vi "Test Copy.vi"(8 "error in (no error)":errorcluster, 11 "Test Case In":refnum<class "01_Image.lvclass">) -> (0 "error out":errorcluster, 3 "Test Case Out":refnum<class "01_Image.lvclass">)   [LabVIEW 2020, in "test.lvlib" / "01_Image.lvclass"]
uses:
  01_Image.lvclass
  C:/Program Files (x86)/National Instruments/LabVIEW 2026/vi.lib/Astemes/LUnit/Test Case.lvclass
  common/Image Size (Integer).ctl
  image/ARGB Colour.ctl
  <vilib>/Astemes/LUnit/Test Case.lvclass/Test Case.ctl
  b8792e11-8542-432e-a0d5-9a7d61cf02c7.vi
  image/New Image (ARGB Preallocated).vi
  image/New Image (Greyscale Preallocated).vi
  image/Copy Image (Greyscale).vi
  4993e8ee-a06a-463a-9684-69129f64d5ce.vi
  image/Copy Image (ARGB).vi
  b39dd01c-c990-4813-b992-e0f28e57d61a.vi
  image/Copy Image (ARGB with Greyscale Mask).vi
  547d0f42-e6d8-4a09-97b6-da1091ed9acb.vi
  image/Copy Image (Greyscale with Mask).vi
  ad9f36d4-cc3b-401b-ad87-e6b842f4a90a.vi
  image/Copy Image (ARGB with ARGB Mask).vi
  53ef6583-9edd-4501-a958-4adbe55cf346.vi
  image/New Image (ARGB Preallocated).vi/3321fa97-f432-4e1e-8db9-a0df79aed21b.vi
  image/ARGB Colour to U32 Pixel Value.vi
  image/New Image (Greyscale Preallocated).vi/6598b9e0-8a08-46f5-91fd-ca1b87217137.vi
  image/Copy Image (Greyscale).vi/c92252ab-1097-45af-a449-7a3c8cf05290.vi
  <vilib>/Astemes/LUnit/Core/LUnit Test Case/Private/Append Pass Result.vi
  <vilib>/Astemes/LUnit/Core/LUnit Test Case/Private/Append Fail Result.vi
  4993e8ee-a06a-463a-9684-69129f64d5ce.vi/9c5d11cd-9439-4240-a1ee-d9baace9c924.vi
  image/Copy Image (ARGB).vi/d58821cd-5760-454c-8714-6bb79b1811ae.vi
  b39dd01c-c990-4813-b992-e0f28e57d61a.vi/9c5d11cd-9439-4240-a1ee-d9baace9c924.vi
  image/Copy Image (ARGB with Greyscale Mask).vi/327a14ae-2acc-4952-87c0-fab6c3cd3da3.vi
  547d0f42-e6d8-4a09-97b6-da1091ed9acb.vi/9c5d11cd-9439-4240-a1ee-d9baace9c924.vi
  image/Copy Image (Greyscale with Mask).vi/1519c485-f8d8-4564-b4f6-4c035770646f.vi
  ad9f36d4-cc3b-401b-ad87-e6b842f4a90a.vi/9c5d11cd-9439-4240-a1ee-d9baace9c924.vi
  image/Copy Image (ARGB with ARGB Mask).vi/3b1fb24f-4521-4d3d-a8b9-ed3d08148c99.vi
  53ef6583-9edd-4501-a958-4adbe55cf346.vi/9c5d11cd-9439-4240-a1ee-d9baace9c924.vi
  <vilib>/Astemes/LUnit/Core/LUnit Test Case/Private/Run In UI.vi
  <vilib>/Utility/error.llb/Clear Errors.vi
  <vilib>/Utility/error.llb/Error Cluster From Error Code.vi
  image/image.lvlib
  common/common.lvlib
  <vilib>/Astemes/LUnit/Test Case.lvclass
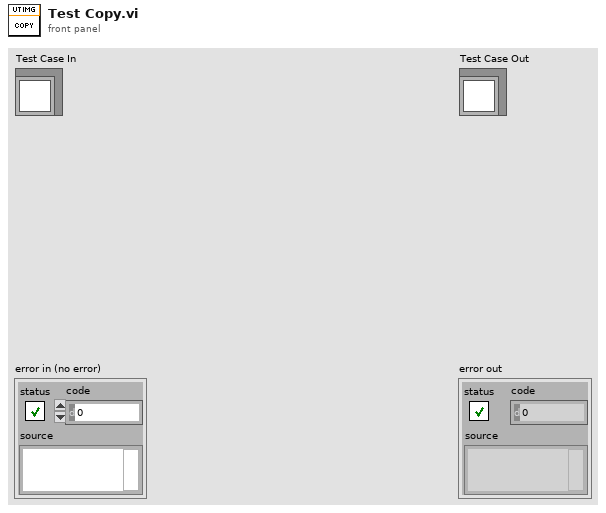
[diagram p1: front panel]
types:
  T1 = typedef "image.lvlib/ARGB Colour.ctl" = cluster{"Alpha":u8, "RGB":u32}
  T2 = typedef "common.lvlib/Image Size (Integer).ctl" = cluster{"Width":u16, "Height":u16}
  T3 = enum16{"ARGB", "Greyscale", "ARGB with Greyscale Mask", "ARGB with ARGB Mask", "Greyscale with Mask"}
  T4 = typedef "image.lvlib/ARGB Image.ctl" = refnum<data-value>
  T5 = typedef "image.lvlib/Greyscale Image.ctl" = refnum<data-value>
  T6 = enum16{"ARGB", "Greyscale", "ARGB with Greyscale Mask", "ARGB with ARGB Mask", "Greyscale with Mask"}[]
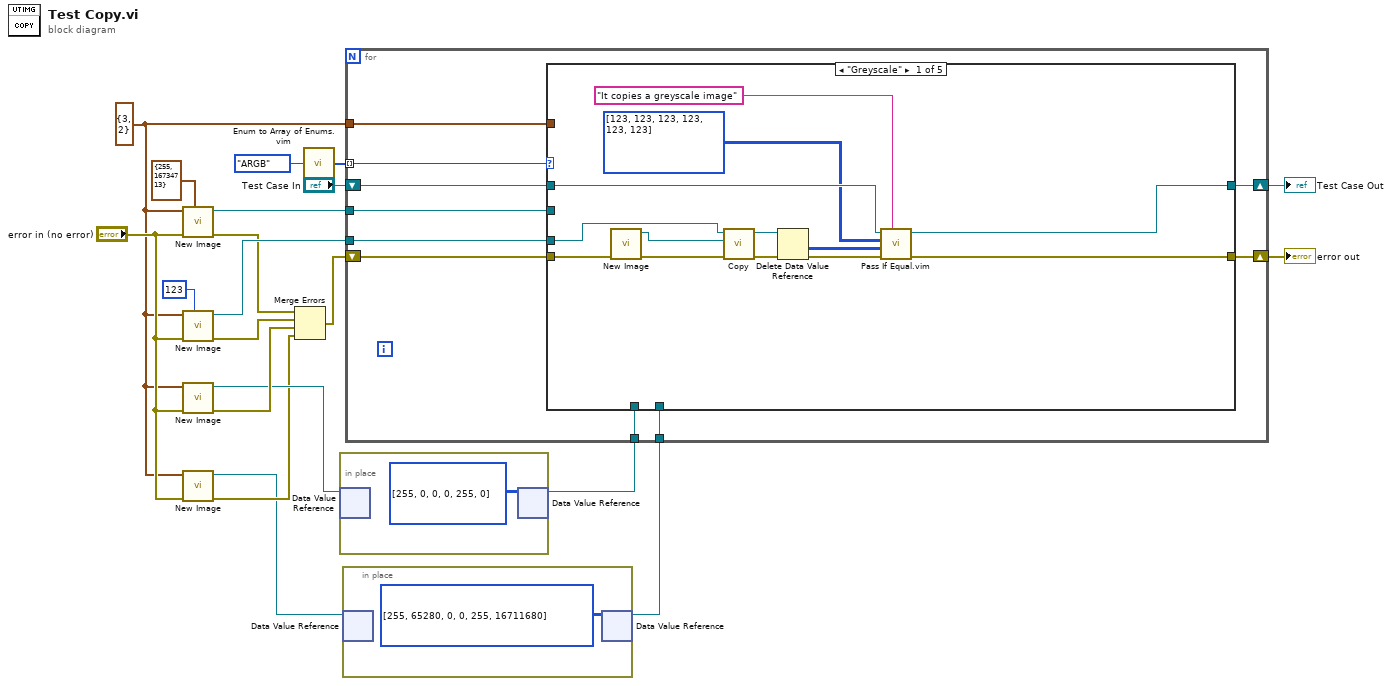
[diagram p0: block diagram]
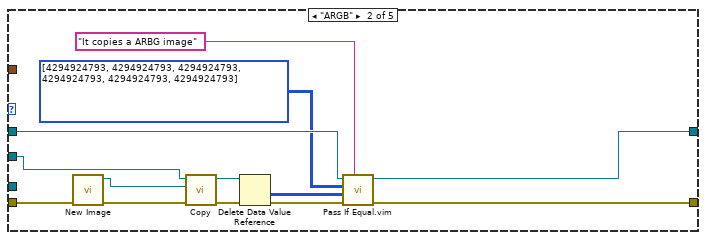
[diagram p2: hidden frame]
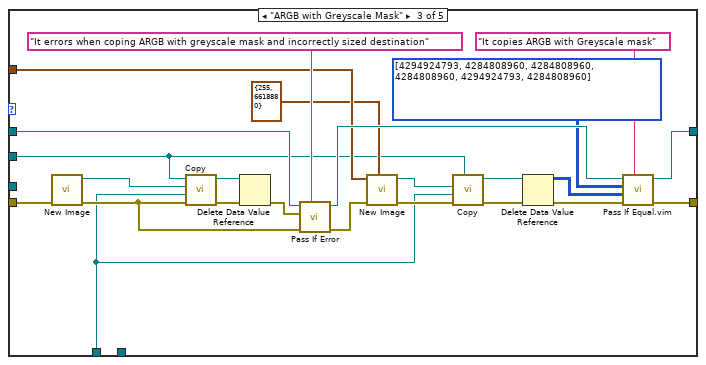
[diagram p3: hidden frame]
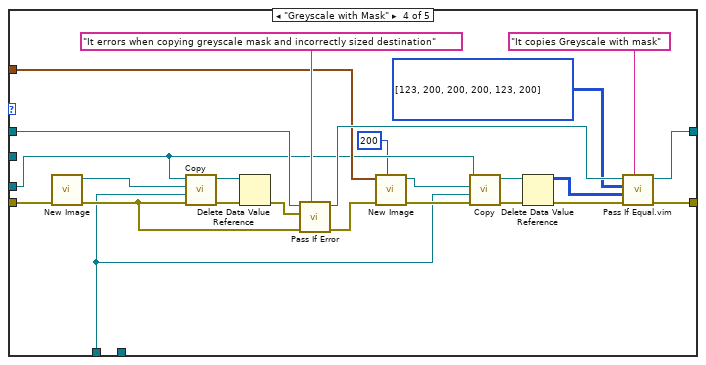
[diagram p4: hidden frame]
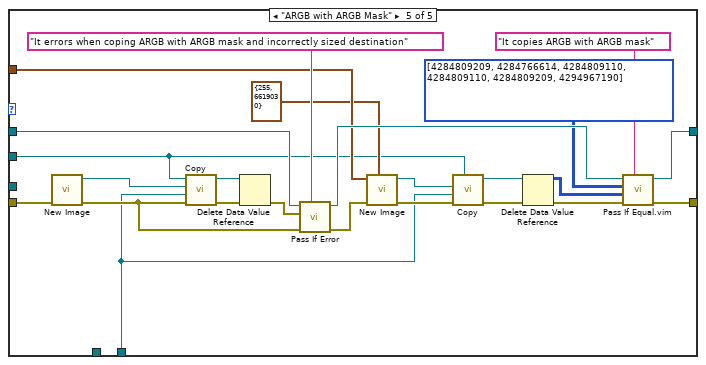
[diagram p5: hidden frame]
diagram:
  w4 = T2 {"Width"=3, "Height"=2} ("Preallocated Image Size (Default: 0,0)")
  n1 = call-poly "New Image.vi"("Colour (Default: Black)"=T1 {"Alpha"=255, "RGB"=16734713}, "error in (no error)"="error in (no error)", "Preallocated Image Size (Default: 0,0)"=w4) -> ("error out"=w13:errorcluster, "ARGB Image"=w14:T4)  [unwired: 7 in]
  n2 = call-poly "New Image.vi"("Value (Default: 0)"=u8 123, "error in (no error)"="error in (no error)", "Preallocated Image Size (Default 0,0)"=w4) -> ("error out"=w12:errorcluster, "Greyscale Image"=w15:T5)  [unwired: 7 in]
  n3 = call-poly "New Image.vi"("error in (no error)"="error in (no error)", "Preallocated Image Size (Default 0,0)"=w4) -> ("error out"=w8:errorcluster, "Greyscale Image"=w7:T5)  [unwired: 8 in]
  n4 = call-poly "New Image.vi"("error in (no error)"="error in (no error)", "Preallocated Image Size (Default: 0,0)"=w4) -> ("error out"=w3:errorcluster, "ARGB Image"=w2:T4)  [unwired: 8 in]
  n5 = Merge Errors(w13, w12, w8, w3) -> (w11:errorcluster)
  n6 = call "Enum to Array of Enums.vim"("enum"=T3."ARGB") -> ("array of enums"=w16:T6)
  n7 = in-place {
    n8 = in-place-dvr #1(w7) -> ()  [unwired: 2 out]
    n9 = in-place-dvr #1(u8[][] [[255, 0, 0], [0, 255, 0]] ("data value")) -> (w6:T5)  [unwired: 1 out]
  }
  n10 = in-place {
    n11 = in-place-dvr #2(w2) -> ()  [unwired: 2 out]
    n12 = in-place-dvr #2(u32[][] [[255, 65280, 0], [0, 255, 16711680]] ("data value")) -> (w1:T4)  [unwired: 1 out]
  }
  n13 = for {
    shift-right: [w31] -> w19
    shift-left: "Test Case In" -> [w32]
    shift-right: [w29] -> w18
    shift-left: w11 -> [w30]
    tunnel: w16 -> [w28] mode=indexing
    tunnel: w15 -> [w27]
    tunnel: w14 -> [w26]
    tunnel: w6 -> [w25]
    tunnel: w4 -> [w24]
    tunnel: w1 -> [w23]
    n14 = case shown="\"Greyscale\"" w28 {
      tunnel: w32 -> [w45 w58 w74 w98 w122]
      tunnel: [w44 w57 w82 w106 w130] -> w31
      tunnel: w30 -> [w40 w54 w79 w103 w127]
      tunnel: [w43 w56 w81 w105 w129] -> w29
      tunnel: w27 -> [w42 _ _ w84 _]
      tunnel: w26 -> [_ w47 w63 _ w112]
      tunnel: w25 -> [_ _ w64 w89 _]
      tunnel: w24 -> [_ _ w66 w90 w114]
      tunnel: w23 -> [_ _ _ _ w109]
      frame "Greyscale" {
        n15 = call-poly "New Image.vi"("error in (no error)"=w40) -> ("error out"=w39:errorcluster, "Greyscale Image"=w38:T5)  [unwired: 9 in]
        n16 = call-poly "Copy.vi"("error in (no error)"=w39, "Greyscale Image Destination in"=w38, "Greyscale Image Source in"=w42) -> ("error out"=w41:errorcluster, "Greyscale Image Destination"=w36:T5)  [unwired: 7 in]
        n17 = Delete Data Value Reference(data value reference=w36, error in=w41) -> (data value=w35:u8[][], error out=w37:errorcluster)
        n18 = call "Pass If Equal.vim"("Description"="It copies a greyscale image", "error in (no error)"=w37, "Actual"=w35, "Expected"=u8[][] [[123, 123, 123], [123, 123, 123]] ("data value"), "LUnit Test Case In"=w45) -> ("error out"=w43:errorcluster, "LUnit Test Case Out"=w44:refnum<class "01_Image.lvclass">)  [unwired: 5 in]
      }
      frame "ARGB" {
        n19 = call-poly "New Image.vi"("error in (no error)"=w54) -> ("error out"=w53:errorcluster, "ARGB Image"=w52:T4)  [unwired: 9 in]
        n20 = call-poly "Copy.vi"("error in (no error)"=w53, "ARGB Image Destination in"=w52, "ARGB Image Source in"=w47) -> ("error out"=w55:errorcluster, "ARGB Image Destination"=w50:T4)  [unwired: 7 in]
        n21 = Delete Data Value Reference(data value reference=w50, error in=w55) -> (data value=w49:u32[][], error out=w51:errorcluster)
        n22 = call "Pass If Equal.vim"("Description"="It copies a ARBG image", "error in (no error)"=w51, "Actual"=w49, "Expected"=u32[][] [[4294924793, 4294924793, 4294924793], [4294924793, 4294924793, 4294924793]] ("data value"), "LUnit Test Case In"=w58) -> ("error out"=w56:errorcluster, "LUnit Test Case Out"=w57:refnum<class "01_Image.lvclass">)  [unwired: 5 in]
      }
      frame "ARGB with Greyscale Mask" {
        n23 = call-poly "New Image.vi"("error in (no error)"=w79) -> ("error out"=w75:errorcluster, "ARGB Image"=w78:T4)  [unwired: 9 in]
        n24 = call-poly "Copy.vi"("error in (no error)"=w75, "Greyscale Image Mask in"=w64, "ARGB Image Destination in"=w78, "ARGB Image Source in"=w63) -> ("error out"=w80:errorcluster, "ARGB Image Destination"=w77:T4)  [unwired: 6 in]
        n25 = Delete Data Value Reference(data value reference=w77, error in=w80) -> (error out=w76:errorcluster)  [unwired: 1 out]
        n26 = call <vilib>:"Pass If Error.vi"("Description"="It errors when coping ARGB with greyscale mask and incorrectly sized destination", "error in (no error)"=w75, "Assert error"=w76, "LUnit Test Case In"=w74) -> ("error out"=w68:errorcluster, "LUnit Test Case Out"=w67:refnum<class "01_Image.lvclass">)  [unwired: 6 in]
        n27 = call-poly "New Image.vi"("Colour (Default: Black)"=T1 {"Alpha"=255, "RGB"=6618880}, "error in (no error)"=w68, "Preallocated Image Size (Default: 0,0)"=w66) -> ("error out"=w72:errorcluster, "ARGB Image"=w70:T4)  [unwired: 7 in]
        n28 = call-poly "Copy.vi"("error in (no error)"=w72, "Greyscale Image Mask in"=w64, "ARGB Image Destination in"=w70, "ARGB Image Source in"=w63) -> ("error out"=w69:errorcluster, "ARGB Image Destination"=w71:T4)  [unwired: 6 in]
        n29 = Delete Data Value Reference(data value reference=w71, error in=w69) -> (data value=w61:u32[][], error out=w62:errorcluster)
        n30 = call "Pass If Equal.vim"("Description"="It copies ARGB with Greyscale mask", "error in (no error)"=w62, "Actual"=w61, "Expected"=u32[][] [[4294924793, 4284808960, 4284808960], [4284808960, 4294924793, 4284808960]] ("data value"), "LUnit Test Case In"=w67) -> ("error out"=w81:errorcluster, "LUnit Test Case Out"=w82:refnum<class "01_Image.lvclass">)  [unwired: 5 in]
      }
      frame "Greyscale with Mask" {
        n31 = call-poly "New Image.vi"("error in (no error)"=w103) -> ("error out"=w99:errorcluster, "Greyscale Image"=w102:T5)  [unwired: 9 in]
        n32 = call-poly "Copy.vi"("error in (no error)"=w99, "Greyscale Image Mask in"=w89, "Greyscale Image Destination in"=w102, "Greyscale Image Source in"=w84) -> ("error out"=w104:errorcluster, "Greyscale Image Destination"=w101:T5)  [unwired: 6 in]
        n33 = Delete Data Value Reference(data value reference=w101, error in=w104) -> (error out=w100:errorcluster)  [unwired: 1 out]
        n34 = call <vilib>:"Pass If Error.vi"("Description"="It errors when copying greyscale mask and incorrectly sized destination", "error in (no error)"=w99, "Assert error"=w100, "LUnit Test Case In"=w98) -> ("error out"=w92:errorcluster, "LUnit Test Case Out"=w91:refnum<class "01_Image.lvclass">)  [unwired: 6 in]
        n35 = call-poly "New Image.vi"("Value (Default: 0)"=u8 200, "error in (no error)"=w92, "Preallocated Image Size (Default 0,0)"=w90) -> ("error out"=w96:errorcluster, "Greyscale Image"=w94:T5)  [unwired: 7 in]
        n36 = call-poly "Copy.vi"("error in (no error)"=w96, "Greyscale Image Mask in"=w89, "Greyscale Image Destination in"=w94, "Greyscale Image Source in"=w84) -> ("error out"=w93:errorcluster, "Greyscale Image Destination"=w95:T5)  [unwired: 6 in]
        n37 = Delete Data Value Reference(data value reference=w95, error in=w93) -> (data value=w87:u8[][], error out=w88:errorcluster)
        n38 = call "Pass If Equal.vim"("Description"="It copies Greyscale with mask", "error in (no error)"=w88, "Actual"=w87, "Expected"=u8[][] [[123, 200, 200], [200, 123, 200]] ("data value"), "LUnit Test Case In"=w91) -> ("error out"=w105:errorcluster, "LUnit Test Case Out"=w106:refnum<class "01_Image.lvclass">)  [unwired: 5 in]
      }
      frame "ARGB with ARGB Mask" {
        n39 = call-poly "New Image.vi"("error in (no error)"=w127) -> ("error out"=w123:errorcluster, "ARGB Image"=w126:T4)  [unwired: 9 in]
        n40 = call-poly "Copy.vi"("error in (no error)"=w123, "ARGB Image Mask in"=w109, "ARGB Image Destination in"=w126, "ARGB Image Source in"=w112) -> ("error out"=w128:errorcluster, "ARGB Image Destination"=w125:T4)  [unwired: 6 in]
        n41 = Delete Data Value Reference(data value reference=w125, error in=w128) -> (error out=w124:errorcluster)  [unwired: 1 out]
        n42 = call <vilib>:"Pass If Error.vi"("Description"="It errors when coping ARGB with ARGB mask and incorrectly sized destination", "error in (no error)"=w123, "Assert error"=w124, "LUnit Test Case In"=w122) -> ("error out"=w116:errorcluster, "LUnit Test Case Out"=w115:refnum<class "01_Image.lvclass">)  [unwired: 6 in]
        n43 = call-poly "New Image.vi"("Colour (Default: Black)"=T1 {"Alpha"=255, "RGB"=6619030}, "error in (no error)"=w116, "Preallocated Image Size (Default: 0,0)"=w114) -> ("error out"=w120:errorcluster, "ARGB Image"=w118:T4)  [unwired: 7 in]
        n44 = call-poly "Copy.vi"("error in (no error)"=w120, "ARGB Image Mask in"=w109, "ARGB Image Destination in"=w118, "ARGB Image Source in"=w112) -> ("error out"=w117:errorcluster, "ARGB Image Destination"=w119:T4)  [unwired: 6 in]
        n45 = Delete Data Value Reference(data value reference=w119, error in=w117) -> (data value=w108:u32[][], error out=w111:errorcluster)
        n46 = call "Pass If Equal.vim"("Description"="It copies ARGB with ARGB mask", "error in (no error)"=w111, "Actual"=w108, "Expected"=u32[][] [[4284809209, 4284766614, 4284809110], [4284809110, 4284809209, 4294967190]] ("data value"), "LUnit Test Case In"=w115) -> ("error out"=w129:errorcluster, "LUnit Test Case Out"=w130:refnum<class "01_Image.lvclass">)  [unwired: 5 in]
      }
    }
  }
  "error out" <- w18
  "Test Case Out" <- w19
